vi "Pool.Create.vi"(7 "FIFO Debug Flags":refnum<class "FIFO Flags.lvclass">, 8 "error in (no error)":errorcluster, 10 "number of elements":u32, 11 "Pool type":refnum<class "Pool.lvclass">) -> (0 "error out":errorcluster, 3 "Pool":refnum<class "Pool.lvclass">)   [LabVIEW 2017, in "DSF.Engine.lvlib" / "Pool.lvclass"]
uses:
  Pool.lvclass
  Debug/FIFO Flags.lvclass
  Pool.lvclass/Pool.ctl
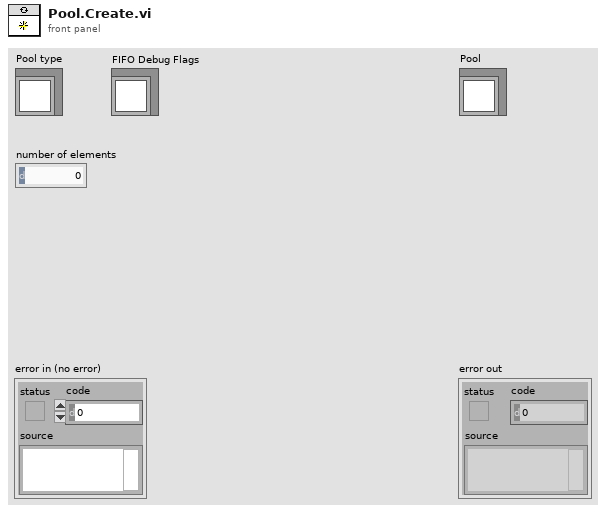
[diagram p1: front panel]
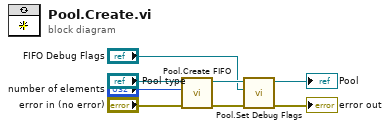
[diagram p0: block diagram]
diagram:
  n1 = call "Pool.Create FIFO.vi"("error in (no error)"="error in (no error)", "number of elements"="number of elements", "Pool in"="Pool type") -> ("error out"=→"error out":errorcluster, "Pool out"=w4:refnum<class "Pool.lvclass">)  [unwired: 7 in]
  n2 = call "Pool.Set Debug Flags.vi"("FIFO Debug Flags"="FIFO Debug Flags", "Pool in"=w4) -> ("Pool out"=→"Pool":refnum<class "Pool.lvclass">)  [unwired: 9 in]
